vi "Sgl_to_Half_Prec.vi"(5 "SGL":sgl) -> (2 "Half Precision Floating Point":u16 format="%016b")   [LabVIEW 2014]
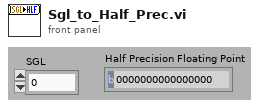
[diagram p1: front panel]
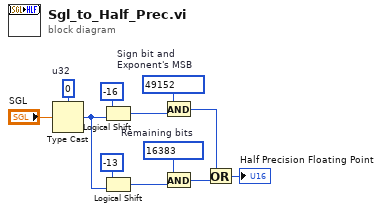
[diagram p0: block diagram]
diagram:
  w5 = u32 0  # u32
  w8 = u32 16383  # Remaining bits
  w11 = u32 49152  # Sign bit and Exponent's MSB
  n1 = Type Cast(type=w5, x="SGL") -> (*(type *) &x=w2:u32)
  n2 = Logical Shift(y=-16, x=w2) -> (x << y=w1:u32)
  n3 = Logical Shift(y=-13, x=w2) -> (x << y=w9:u32)
  n4 = And(x=w11, y=w1) -> (x .and. y?=w6:u32)
  n5 = And(x=w8, y=w9) -> (x .and. y?=w7:u32)
  n6 = Or(x=w6, y=w7) -> (x .or. y?=→"Half Precision Floating Point":u32)
